vi "Kaelus SWI Preset.vi"(7 "Kaelus SWI":T4, 8 "error in (no error)":errorcluster, 11 "DAQmx Dev Name (SWModule)":string) -> (0 "error out":errorcluster, 3 "DAQmx Dev Name (SWModule)":string, 5 "SWI Position":T1)   [LabVIEW 2011]
uses:
  TypeDefs/Kaelus SWI Instrument Info.ctl
  TypeDefs/Kaelus SWI Position.ctl
  PIM/BPIM Web Engine/LIB/MODULES/SW Module/SW Tx Positions.ctl
  PIM/BPIM Web Engine/LIB/MODULES/SW Module/SW Rx Positions.ctl
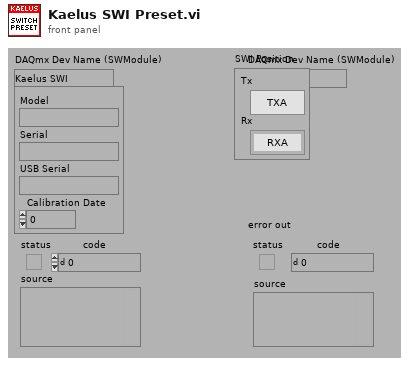
[diagram p1: front panel]
types:
  T1 = typedef "Kaelus SWI Position.ctl" = cluster{"Tx":T2, "Rx":T3}
  T2 = typedef "SW Tx Positions.ctl" = enum16{"TXA", "TXB", "TXC"}
  T3 = typedef "SW Rx Positions.ctl" = enum16{"RXA", "RXB", "RXC", "RXD", "RXE", "RXF"}
  T4 = typedef "Kaelus SWI Instrument Info.ctl" = cluster{"Model":string, "Serial":string, "USB Serial":string, "Calibration Date":dbl}
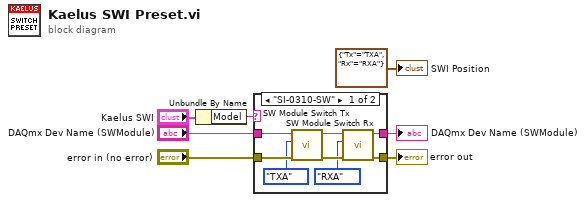
[diagram p0: block diagram]
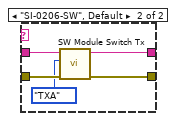
[diagram p2: hidden frame]
diagram:
  n1 = Unbundle By Name("Kaelus SWI") -> ("Model"=w6:string)
  n2 = case shown="\"SI-0310-SW\"" w6 {
    tunnel: "error in (no error)" -> [w12 w17]
    tunnel: [w11 w16] -> w1
    tunnel: "DAQmx Dev Name (SWModule)" -> [w10 w15]
    tunnel: [w10 w15] -> w2
    frame "SI-0310-SW" {
      n3 = call "SW Module Switch Tx.vi"("error in (no error)"=w12, "Tx Position"=SW_Tx_Positions."TXA", "SW Dmx Name"=w10) -> ("error out"=w13:errorcluster)  [unwired: 8 out]
      n4 = call "SW Module Switch Rx.vi"("error in (no error)"=w13, "Rx Position"=SW_Rx_Positions."RXA", "SW Dmx Name"=w10) -> ("error out"=w11:errorcluster)  [unwired: 8 out]
    }
    frame "SI-0206-SW", Default {
      n5 = call "SW Module Switch Tx.vi"("error in (no error)"=w17, "Tx Position"=SW_Tx_Positions."TXA", "SW Dmx Name"=w15) -> ("error out"=w16:errorcluster)  [unwired: 8 out]
    }
  }
  "error out" <- w1
  "DAQmx Dev Name (SWModule)" <- w2
  "SWI Position" <- T1 {"Tx"=enum."TXA", "Rx"=enum."RXA"} ("SWI Position")
